vi "Motor_Controller.vi"(0 "error in (no error)":errorcluster, 7 "motorSelect":enum16{"Motor A", "Motor B"}(ring), 9 "direction":enum16{"Forward", "Backward"}(ring), 11 "stopMotors":bool) -> (4 "error out":errorcluster)   [LabVIEW 2016]
uses:
  <vilib>/myRIO/Instrument Drivers/Onboard IO/DIO/typedefs/DIO Reference.ctl
  <vilib>/myRIO/Common/Instrument Driver Framework/Utilities/typedefs/myRIO Generic Hardware Reference.ctl
  <vilib>/myRIO/Common/Instrument Driver Framework/Utilities/typedefs/Hardware Version Enum.ctl
  <vilib>/myRIO/Common/Instrument Driver Framework/Utilities/typedefs/myRIO v1.0 Reference.ctl
  <vilib>/myRIO/Common/Instrument Driver Framework/Utilities/typedefs/Generic FPGA Reference.ctl
  <vilib>/myRIO/Common/Instrument Driver Framework/myRIO v1.0/DIO/typedefs/DIO Channels List.ctl
  <vilib>/myRIO/Common/Instrument Driver Framework/myRIO v1.0/DIO/typedefs/DIO Channels Enum.ctl
  <vilib>/userdefined/High Color/nirio_resource_hc.ctl
  <vilib>/myRIO/Common/Instrument Driver Framework/Utilities/vis/Is FPGA Ref Available.vi
  <vilib>/myRIO/Common/Instrument Driver Framework/roboRIO v1.0/DIO/vis/roboRIO v1.0 Open DIO.vi
  <vilib>/myRIO/Instrument Drivers/Onboard IO/DIO/vis/Write.vi
  <vilib>/myRIO/Common/Instrument Driver Framework/Utilities/vis/Validate Channels.vi
  <vilib>/myRIO/Common/Instrument Driver Framework/roboRIO v1.0/DIO/vis/roboRIO v1.0 Reserve DIO.vi
  <vilib>/myRIO/Common/Instrument Driver Framework/roboRIO v1.0/DIO/vis/roboRIO v1.0 Build MUX Configuration DIO.vi
  <vilib>/myRIO/Common/Instrument Driver Framework/roboRIO v1.0/Resource Manager/vis/roboRIO v1.0 Reserve Channel List.vi
  <vilib>/myRIO/Common/Instrument Driver Framework/roboRIO v1.0/Resource Manager/vis/roboRIO v1.0 Create Configuration List.vi
  <vilib>/myRIO/Common/Instrument Driver Framework/roboRIO v1.0/Resource Manager/vis/roboRIO v1.0 Reserve Channel.vi
  <vilib>/myRIO/Common/Instrument Driver Framework/roboRIO v1.0/Resource Manager/vis/roboRIO v1.0 Unreserve Channel.vi
  <vilib>/myRIO/Common/Instrument Driver Framework/roboRIO v1.0/Resource Manager/vis/roboRIO v1.0 Build Mutex Name.vi
  <vilib>/Utility/VariantDataType/GetNumericInfo.vi
  builds/UnicornMain/UnicornRIO1/ROS for LabVIEW/home/lvuser/natinst/bin/vi.lib/Utility/error.llb/Error Cluster From Error Code.vi
  <vilib>/myRIO/Common/Instrument Driver Framework/roboRIO v1.0/roboRIO v1.0 Open.vi
  <vilib>/myRIO/Common/Instrument Driver Framework/Utilities/vis/IO Manager.vi
  <vilib>/myRIO/Common/Instrument Driver Framework/Utilities/vis/Configuration Manager.vi
  <vilib>/myRIO/Common/Instrument Driver Framework/roboRIO v1.0/Resource Manager/vis/roboRIO v1.0 Configure IO.vi
  <vilib>/myRIO/Common/Instrument Driver Framework/myRIO v1.0/myRIO v1.0 Close.vi
  <vilib>/myRIO/Common/Instrument Driver Framework/roboRIO v1.0/DIO/vis/roboRIO v1.0 Write DIO.vi
  <vilib>/myRIO/Express VI/Onboard IO/DO/DO Express VI.xnode
  <vilib>/myRIO/Instrument Drivers/Onboard IO/DIO/vis/myRIO DIO Open.xnode
  <vilib>/myRIO/Instrument Drivers/Onboard IO/DIO/DIO.lvlib
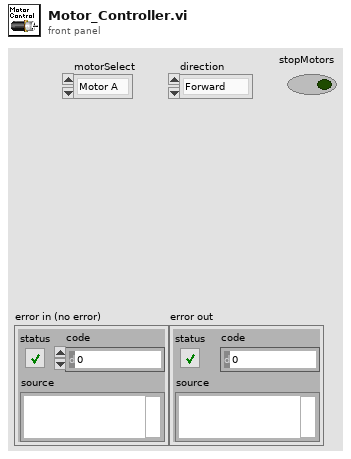
[diagram p1: front panel]
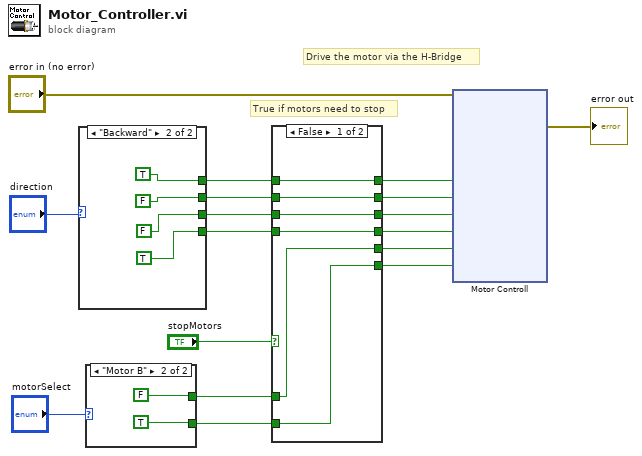
[diagram p0: block diagram]
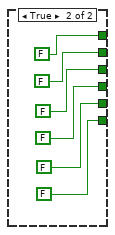
[diagram p2: hidden frame]
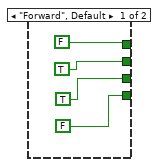
[diagram p3: hidden frame]
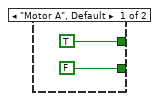
[diagram p4: hidden frame]
diagram:
  # "True if motors need to stop"
  # "Drive the motor via the H-Bridge"
  n1 = case shown="\"Backward\"" "direction" {
    tunnel: [FALSE TRUE] -> w10
    tunnel: [TRUE FALSE] -> w11
    tunnel: [TRUE FALSE] -> w12
    tunnel: [FALSE TRUE] -> w13
    frame "Forward", Default {
    }
    frame "Backward" {
    }
  }
  n2 = case shown="\"Motor B\"" "motorSelect" {
    tunnel: [TRUE FALSE] -> w15
    tunnel: [FALSE TRUE] -> w14
    frame "Motor A", Default {
    }
    frame "Motor B" {
    }
  }
  n3 = case shown="False" "stopMotors" {
    tunnel: w15 -> [w31 _]
    tunnel: w14 -> [w30 _]
    tunnel: w13 -> [w32 _]
    tunnel: w12 -> [w33 _]
    tunnel: w11 -> [w34 _]
    tunnel: w10 -> [w35 _]
    tunnel: [w35 FALSE] -> w5
    tunnel: [w34 FALSE] -> w4
    tunnel: [w33 FALSE] -> w2
    tunnel: [w32 FALSE] -> w1
    tunnel: [w31 FALSE] -> w3
    tunnel: [w30 FALSE] -> w6
    frame False {
    }
    frame True {
    }
  }
  n4 = xnode "Motor Controll"("IN1 (B/DIO1 (Pin 13))"=w5, "IN2 (B/DIO2 (Pin 15))"=w4, "IN3 (B/DIO3 (Pin 17))"=w2, "IN4 (B/DIO4 (Pin 19))"=w1, "ENABLE A (B/DIO0 (Pin 11))"=w3, "ENABLE B (B/DIO5 (Pin 21))"=w6, "error in (no error)"="error in (no error)") -> ("error out"=→"error out":errorcluster)
